vi "Move-Axis-Sync.vi"(0 "x mm":dbl, 1 "Settings":T1, 2 "Speed X":i32) -> ()   [LabVIEW 2017]
uses:
  Settings/Settings-Control.ctl
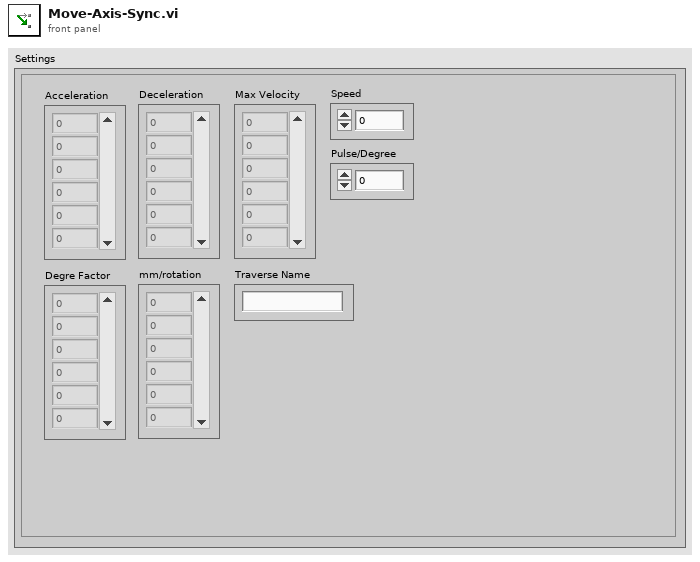
[diagram p1: front panel]
types:
  T1 = typedef "Settings-Control.ctl" = cluster{"Acceleration":dbl[], "Deceleration":dbl[], "Max Velocity":dbl[], "Speed":dbl, "Pulse/Degree":dbl, "Degre Factor":dbl[], "mm/rotation":dbl[], "Traverse Name":string}
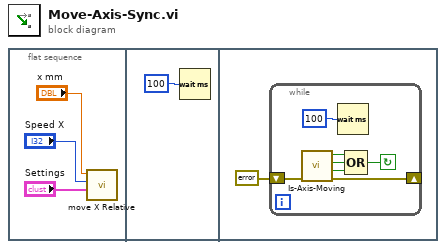
[diagram p0: block diagram]
diagram:
  n1 = flat-sequence {
    frame #0 {
      n2 = call "move X Relative.vi"("Settings"="Settings", "Speed X"="Speed X", "x mm"="x mm") -> ()  [unwired: 9 in]
    }
    frame #1 {
      n3 = Wait (ms)(milliseconds to wait=u32 100) -> ()  [unwired: 1 out]
    }
    frame #2 {
      n4 = while {
        shift-right: [w10] -> _
        shift-left: errorcluster {"status"=FALSE, "code"=0, "source"=""} ("error out") -> [w11]
        stop <- w6 continue-if-true
        n5 = call "Is-Axis-Moving.vi"("error in"=w11) -> ("error out"=w10:errorcluster, "Z"=w7:bool, "Y"=w8:bool, "X"=w9:bool)  [unwired: 7 in]
        n6 = Wait (ms)(milliseconds to wait=u32 100) -> ()  [unwired: 1 out]
        n7 = Compound Arithmetic op=OR(w9, w8, w7) -> (w6:bool)
      }
    }
  }
